vi "rs3 set multi options.vi"(4 "laser on/off":bool, 6 "autoexposure":bool, 7 "Laser power, mW (0-360)":sgl, 8 "error in (no error)":errorcluster, 9 "Gain(16-248)":sgl=16.0, 10 "Exposure, us":sgl=33000.0, 11 "Sensor in":u64) -> (0 "error out":errorcluster, 2 "Set Option error":string, 3 "Sensor out":u64)   [LabVIEW 2017, in "libRealSense3.lvlib"]
doc: "Sets the multiple device options. \n \nINPUT:\nExposure The manual exposure of the SENSOR, in microseconds\nGain The gain of the sensor from 16-248. For best results for depth keep this as low as possible\nLaser power The power of the projector in mW.\nLaser on/off Turns projector on/off.\nautoexposure Turns on the autoexplosure function which will automatically adjust gain and exposure. To change the setpoint it is possible to use the VIs that change the ROI (region of intested) as well as the SETPOINT for the autoexposure function. \n \nOutput:\nerror if non-null, receives any error that occurs during this call, otherwise, errors are ignored"
uses:
  <vilib>/addons/RealSense/libRealSense3.lvlib
panel:
  # "RS2_OPTION_BACKLIGHT_COMPENSATION                     , /**< Enable / disable color backlight compensation*/\n    RS2_OPTION_BRIGHTNESS                                 , /**< Color image brightness*/\n    RS2_OPTION_CONTRAST                                   , /**< Color image contrast*/\n    RS2_OPTION_EXPOSURE                                   , /**< Controls exposure time of color camera. Setting any value will disable auto exposure*/\n    RS2_OPTION_GAIN                                       , /**< Color image gain*/\n    RS2_OPTION_GAMMA                                      , /**< Color image gamma setting*/\n    RS2_OPTION_HUE                                        , /**< Color image hue*/\n    RS2_OPTION_SATURATION                                 , /**< Color image saturation setting*/\n    RS2_OPTION_SHARPNESS                                  , /**< Color image sharpness setting*/\n    RS2_OPTION_WHITE_BALANCE                              , /**< Controls white balance of color image. Setting any value will disable auto white balance*/\n    RS2_OPTION_ENABLE_AUTO_EXPOSURE                       , /**< Enable / disable color image auto-exposure*/\n    RS2_OPTION_ENABLE_AUTO_WHITE_BALANCE                  , /**< Enable / disable color image auto-white-balance*/\n    RS2_OPTION_VISUAL_PRESET                              , /**< Provide access to several recommend sets of option presets for the depth camera */\n    RS2_OPTION_LASER_POWER                                , /**< Power of the F200 / SR300 projector, with 0 meaning projector off*/\n    RS2_OPTION_ACCURACY                                   , /**< Set the number of patterns projected per frame. The higher the accuracy value the more patterns projected. Increasing the number of patterns help to achieve better accuracy. Note that this control is affecting the Depth FPS */\n    RS2_OPTION_MOTION_RANGE                               , /**< Motion vs. Range trade-off, with lower values allowing for better motion sensitivity and higher values allowing for better depth range*/\n    RS2_OPTION_FILTER_OPTION                              , /**< Set the filter to apply to each depth frame. Each one of the filter is optimized per the application requirements*/\n    RS2_OPTION_CONFIDENCE_THRESHOLD                       , /**< The confidence level threshold used by the Depth algorithm pipe to set whether a pixel will get a valid range or will be marked with invalid range*/\n    RS2_OPTION_EMITTER_ENABLED                            , /**< Laser Emitter enabled */\n    RS2_OPTION_FRAMES_QUEUE_SIZE                          , /**< Number of frames the user is allowed to keep per stream. Trying to hold-on to more frames will cause frame-drops.*/\n    RS2_OPTION_TOTAL_FRAME_DROPS                          , /**< Total number of detected frame drops from all streams */\n    RS2_OPTION_AUTO_EXPOSURE_MODE                         , /**< Auto-Exposure modes: Static, Anti-Flicker and Hybrid */\n    RS2_OPTION_AUTO_EXPOSURE_ANTIFLICKER_RATE             , /**< Auto-Exposure anti-flicker rate, can be 50 or 60 Hz */\n    RS2_OPTION_ASIC_TEMPERATURE                           , /**< Current Asic Temperature */\n    RS2_OPTION_ERROR_POLLING_ENABLED                      , /**< disable error handling */\n    RS2_OPTION_PROJECTOR_TEMPERATURE                      , /**< Current Projector Temperature */\n    RS2_OPTION_OUTPUT_TRIGGER_ENABLED                     , /**< Enable / disable trigger to be outputed from the camera to any external device on every depth frame */\n    RS2_OPTION_MOTION_MODULE_TEMPERATURE                  , /**< Current Motion-Module Temperature */\n    RS2_OPTION_COUNT                                      , /**< Number of enumeration values. Not a valid input: intended to be used in for-loops. */"
  # "RS3 Set Multi Device Option"
  # "(C) 2017 Intel Corp.,  AGJ"
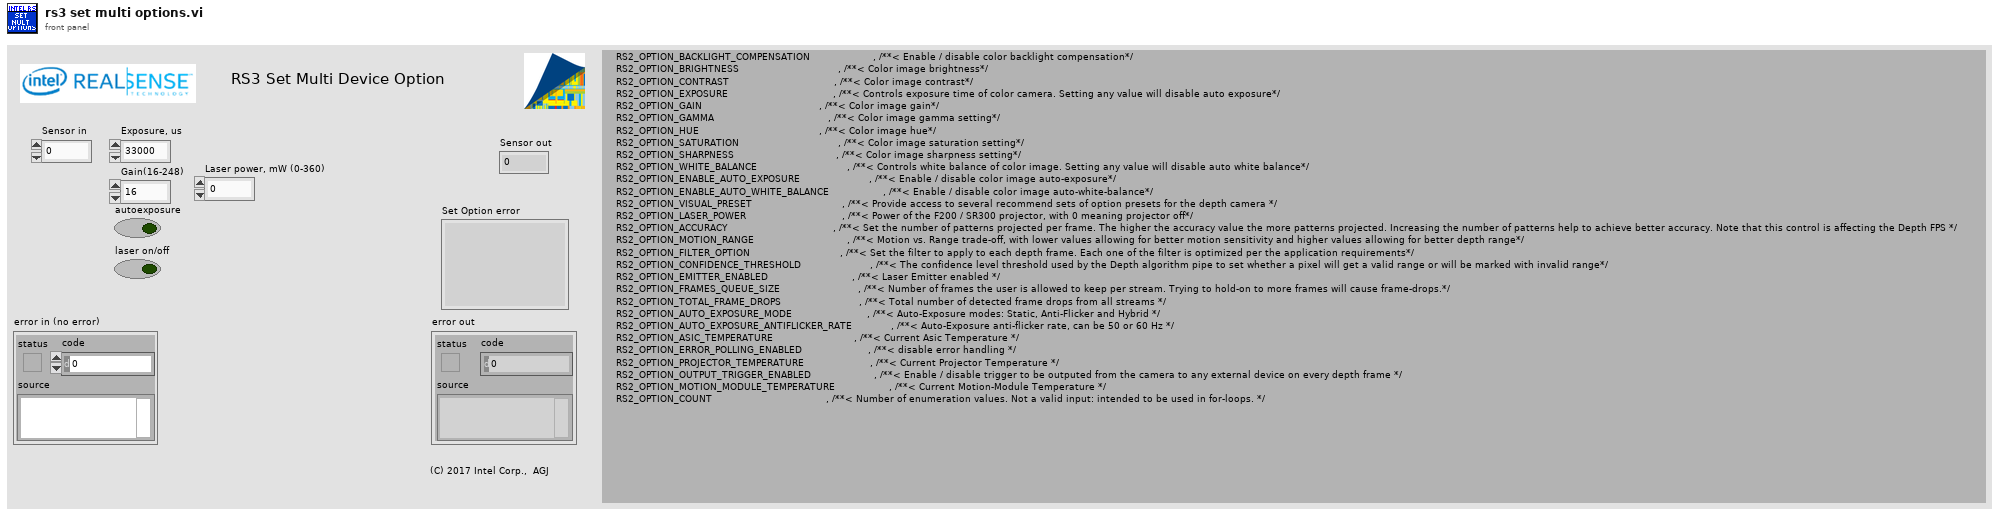
[diagram p1: front panel]
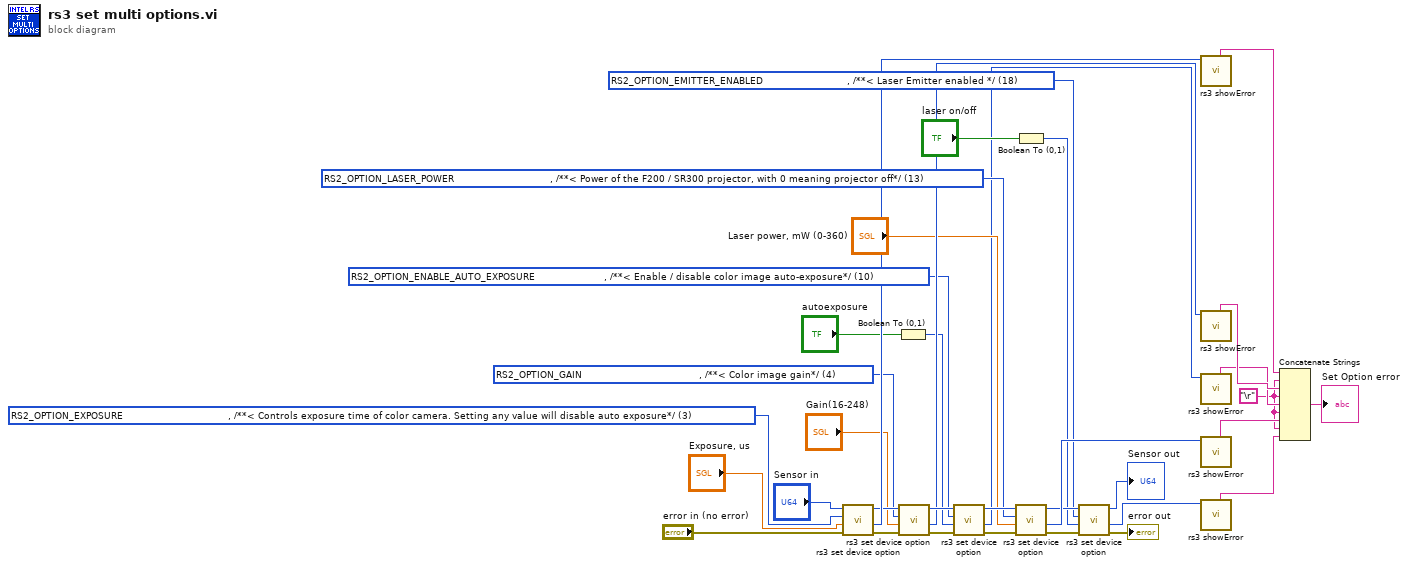
[diagram p0: block diagram]
diagram:
  w2 = u16 10 items=["    RS2_OPTION_BACKLIGHT_COMPENSATION                     , /**< Enable / disable color backlight compensation*/", "    RS2_OPTION_BRIGHTNESS                                 , /**< Color image brightness*/", "    RS2_OPTION_CONTRAST                                   , /**< Color image contrast*/", "    RS2_OPTION_EXPOSURE                                   , /**< Controls exposure time of color camera. Setting any value will disable auto exposure*/", "    RS2_OPTION_GAIN                                       , /**< Color image gain*/", "    RS2_OPTION_GAMMA                                      , /**< Color image gamma setting*/", "    RS2_OPTION_HUE                                        , /**< Color image hue*/", "    RS2_OPTION_SATURATION                                 , /**< Color image saturation setting*/", "    RS2_OPTION_SHARPNESS                                  , /**< Color image sharpness setting*/", "    RS2_OPTION_WHITE_BALANCE                              , /**< Controls white balance of color image. Setting any value will disable auto white balance*/", "    RS2_OPTION_ENABLE_AUTO_EXPOSURE                       , /**< Enable / disable color image auto-exposure*/", "    RS2_OPTION_ENABLE_AUTO_WHITE_BALANCE                  , /**< Enable / disable color image auto-white-balance*/", "    RS2_OPTION_VISUAL_PRESET                              , /**< Provide access to several recommend sets of option presets for the depth camera */", "    RS2_OPTION_LASER_POWER                                , /**< Power of the F200 / SR300 projector, with 0 meaning projector off*/", "    RS2_OPTION_ACCURACY                                   , /**< Set the number of patterns projected per frame. The higher the accuracy value the more patterns projected. Increasing the number of patterns help to achieve better accuracy. Note that this c", "    RS2_OPTION_MOTION_RANGE                               , /**< Motion vs. Range trade-off, with lower values allowing for better motion sensitivity and higher values allowing for better depth range*/", "    RS2_OPTION_FILTER_OPTION                              , /**< Set the filter to apply to each depth frame. Each one of the filter is optimized per the application requirements*/", "    RS2_OPTION_CONFIDENCE_THRESHOLD                       , /**< The confidence level threshold used by the Depth algorithm pipe to set whether a pixel will get a valid range or will be marked with invalid range*/", "    RS2_OPTION_EMITTER_ENABLED                            , /**< Laser Emitter enabled */", "    RS2_OPTION_FRAMES_QUEUE_SIZE                          , /**< Number of frames the user is allowed to keep per stream. Trying to hold-on to more frames will cause frame-drops.*/", "    RS2_OPTION_TOTAL_FRAME_DROPS                          , /**< Total number of detected frame drops from all streams */", "    RS2_OPTION_AUTO_EXPOSURE_MODE                         , /**< Auto-Exposure modes: Static, Anti-Flicker and Hybrid */", "    RS2_OPTION_POWER_LINE_FREQUENCY                       , /**< Power Line Frequency control for anti-flickering Off/50Hz/60Hz/Auto */", "    RS2_OPTION_ASIC_TEMPERATURE                           , /**< Current Asic Temperature */", "    RS2_OPTION_ERROR_POLLING_ENABLED                      , /**< disable error handling */", "    RS2_OPTION_PROJECTOR_TEMPERATURE                      , /**< Current Projector Temperature */", "    RS2_OPTION_OUTPUT_TRIGGER_ENABLED                     , /**< Enable / disable trigger to be outputed from the camera to any external device on every depth frame */", "    RS2_OPTION_MOTION_MODULE_TEMPERATURE                  , /**< Current Motion-Module Temperature */", "    RS2_OPTION_DEPTH_UNITS                                , /**< Number of meters represented by a single depth unit */", "    RS2_OPTION_ENABLE_MOTION_CORRECTION                   , /**< Enable/Disable automatic correction of the motion data */", "    RS2_OPTION_AUTO_EXPOSURE_PRIORITY                     , /**< Allows sensor to dynamically ajust the frame rate depending on lighting conditions */", "    RS2_OPTION_COUNT                                      , /**< Number of enumeration values. Not a valid input: intended to be used in for-loops. */"] ("RS Option")
  w5 = u16 13 items=["    RS2_OPTION_BACKLIGHT_COMPENSATION                     , /**< Enable / disable color backlight compensation*/", "    RS2_OPTION_BRIGHTNESS                                 , /**< Color image brightness*/", "    RS2_OPTION_CONTRAST                                   , /**< Color image contrast*/", "    RS2_OPTION_EXPOSURE                                   , /**< Controls exposure time of color camera. Setting any value will disable auto exposure*/", "    RS2_OPTION_GAIN                                       , /**< Color image gain*/", "    RS2_OPTION_GAMMA                                      , /**< Color image gamma setting*/", "    RS2_OPTION_HUE                                        , /**< Color image hue*/", "    RS2_OPTION_SATURATION                                 , /**< Color image saturation setting*/", "    RS2_OPTION_SHARPNESS                                  , /**< Color image sharpness setting*/", "    RS2_OPTION_WHITE_BALANCE                              , /**< Controls white balance of color image. Setting any value will disable auto white balance*/", "    RS2_OPTION_ENABLE_AUTO_EXPOSURE                       , /**< Enable / disable color image auto-exposure*/", "    RS2_OPTION_ENABLE_AUTO_WHITE_BALANCE                  , /**< Enable / disable color image auto-white-balance*/", "    RS2_OPTION_VISUAL_PRESET                              , /**< Provide access to several recommend sets of option presets for the depth camera */", "    RS2_OPTION_LASER_POWER                                , /**< Power of the F200 / SR300 projector, with 0 meaning projector off*/", "    RS2_OPTION_ACCURACY                                   , /**< Set the number of patterns projected per frame. The higher the accuracy value the more patterns projected. Increasing the number of patterns help to achieve better accuracy. Note that this c", "    RS2_OPTION_MOTION_RANGE                               , /**< Motion vs. Range trade-off, with lower values allowing for better motion sensitivity and higher values allowing for better depth range*/", "    RS2_OPTION_FILTER_OPTION                              , /**< Set the filter to apply to each depth frame. Each one of the filter is optimized per the application requirements*/", "    RS2_OPTION_CONFIDENCE_THRESHOLD                       , /**< The confidence level threshold used by the Depth algorithm pipe to set whether a pixel will get a valid range or will be marked with invalid range*/", "    RS2_OPTION_EMITTER_ENABLED                            , /**< Laser Emitter enabled */", "    RS2_OPTION_FRAMES_QUEUE_SIZE                          , /**< Number of frames the user is allowed to keep per stream. Trying to hold-on to more frames will cause frame-drops.*/", "    RS2_OPTION_TOTAL_FRAME_DROPS                          , /**< Total number of detected frame drops from all streams */", "    RS2_OPTION_AUTO_EXPOSURE_MODE                         , /**< Auto-Exposure modes: Static, Anti-Flicker and Hybrid */", "    RS2_OPTION_POWER_LINE_FREQUENCY                       , /**< Power Line Frequency control for anti-flickering Off/50Hz/60Hz/Auto */", "    RS2_OPTION_ASIC_TEMPERATURE                           , /**< Current Asic Temperature */", "    RS2_OPTION_ERROR_POLLING_ENABLED                      , /**< disable error handling */", "    RS2_OPTION_PROJECTOR_TEMPERATURE                      , /**< Current Projector Temperature */", "    RS2_OPTION_OUTPUT_TRIGGER_ENABLED                     , /**< Enable / disable trigger to be outputed from the camera to any external device on every depth frame */", "    RS2_OPTION_MOTION_MODULE_TEMPERATURE                  , /**< Current Motion-Module Temperature */", "    RS2_OPTION_DEPTH_UNITS                                , /**< Number of meters represented by a single depth unit */", "    RS2_OPTION_ENABLE_MOTION_CORRECTION                   , /**< Enable/Disable automatic correction of the motion data */", "    RS2_OPTION_AUTO_EXPOSURE_PRIORITY                     , /**< Allows sensor to dynamically ajust the frame rate depending on lighting conditions */", "    RS2_OPTION_COUNT                                      , /**< Number of enumeration values. Not a valid input: intended to be used in for-loops. */"] ("RS Option")
  w7 = u16 18 items=["    RS2_OPTION_BACKLIGHT_COMPENSATION                     , /**< Enable / disable color backlight compensation*/", "    RS2_OPTION_BRIGHTNESS                                 , /**< Color image brightness*/", "    RS2_OPTION_CONTRAST                                   , /**< Color image contrast*/", "    RS2_OPTION_EXPOSURE                                   , /**< Controls exposure time of color camera. Setting any value will disable auto exposure*/", "    RS2_OPTION_GAIN                                       , /**< Color image gain*/", "    RS2_OPTION_GAMMA                                      , /**< Color image gamma setting*/", "    RS2_OPTION_HUE                                        , /**< Color image hue*/", "    RS2_OPTION_SATURATION                                 , /**< Color image saturation setting*/", "    RS2_OPTION_SHARPNESS                                  , /**< Color image sharpness setting*/", "    RS2_OPTION_WHITE_BALANCE                              , /**< Controls white balance of color image. Setting any value will disable auto white balance*/", "    RS2_OPTION_ENABLE_AUTO_EXPOSURE                       , /**< Enable / disable color image auto-exposure*/", "    RS2_OPTION_ENABLE_AUTO_WHITE_BALANCE                  , /**< Enable / disable color image auto-white-balance*/", "    RS2_OPTION_VISUAL_PRESET                              , /**< Provide access to several recommend sets of option presets for the depth camera */", "    RS2_OPTION_LASER_POWER                                , /**< Power of the F200 / SR300 projector, with 0 meaning projector off*/", "    RS2_OPTION_ACCURACY                                   , /**< Set the number of patterns projected per frame. The higher the accuracy value the more patterns projected. Increasing the number of patterns help to achieve better accuracy. Note that this c", "    RS2_OPTION_MOTION_RANGE                               , /**< Motion vs. Range trade-off, with lower values allowing for better motion sensitivity and higher values allowing for better depth range*/", "    RS2_OPTION_FILTER_OPTION                              , /**< Set the filter to apply to each depth frame. Each one of the filter is optimized per the application requirements*/", "    RS2_OPTION_CONFIDENCE_THRESHOLD                       , /**< The confidence level threshold used by the Depth algorithm pipe to set whether a pixel will get a valid range or will be marked with invalid range*/", "    RS2_OPTION_EMITTER_ENABLED                            , /**< Laser Emitter enabled */", "    RS2_OPTION_FRAMES_QUEUE_SIZE                          , /**< Number of frames the user is allowed to keep per stream. Trying to hold-on to more frames will cause frame-drops.*/", "    RS2_OPTION_TOTAL_FRAME_DROPS                          , /**< Total number of detected frame drops from all streams */", "    RS2_OPTION_AUTO_EXPOSURE_MODE                         , /**< Auto-Exposure modes: Static, Anti-Flicker and Hybrid */", "    RS2_OPTION_POWER_LINE_FREQUENCY                       , /**< Power Line Frequency control for anti-flickering Off/50Hz/60Hz/Auto */", "    RS2_OPTION_ASIC_TEMPERATURE                           , /**< Current Asic Temperature */", "    RS2_OPTION_ERROR_POLLING_ENABLED                      , /**< disable error handling */", "    RS2_OPTION_PROJECTOR_TEMPERATURE                      , /**< Current Projector Temperature */", "    RS2_OPTION_OUTPUT_TRIGGER_ENABLED                     , /**< Enable / disable trigger to be outputed from the camera to any external device on every depth frame */", "    RS2_OPTION_MOTION_MODULE_TEMPERATURE                  , /**< Current Motion-Module Temperature */", "    RS2_OPTION_DEPTH_UNITS                                , /**< Number of meters represented by a single depth unit */", "    RS2_OPTION_ENABLE_MOTION_CORRECTION                   , /**< Enable/Disable automatic correction of the motion data */", "    RS2_OPTION_AUTO_EXPOSURE_PRIORITY                     , /**< Allows sensor to dynamically ajust the frame rate depending on lighting conditions */", "    RS2_OPTION_COUNT                                      , /**< Number of enumeration values. Not a valid input: intended to be used in for-loops. */"] ("RS Option")
  w13 = u16 4 items=["    RS2_OPTION_BACKLIGHT_COMPENSATION                     , /**< Enable / disable color backlight compensation*/", "    RS2_OPTION_BRIGHTNESS                                 , /**< Color image brightness*/", "    RS2_OPTION_CONTRAST                                   , /**< Color image contrast*/", "    RS2_OPTION_EXPOSURE                                   , /**< Controls exposure time of color camera. Setting any value will disable auto exposure*/", "    RS2_OPTION_GAIN                                       , /**< Color image gain*/", "    RS2_OPTION_GAMMA                                      , /**< Color image gamma setting*/", "    RS2_OPTION_HUE                                        , /**< Color image hue*/", "    RS2_OPTION_SATURATION                                 , /**< Color image saturation setting*/", "    RS2_OPTION_SHARPNESS                                  , /**< Color image sharpness setting*/", "    RS2_OPTION_WHITE_BALANCE                              , /**< Controls white balance of color image. Setting any value will disable auto white balance*/", "    RS2_OPTION_ENABLE_AUTO_EXPOSURE                       , /**< Enable / disable color image auto-exposure*/", "    RS2_OPTION_ENABLE_AUTO_WHITE_BALANCE                  , /**< Enable / disable color image auto-white-balance*/", "    RS2_OPTION_VISUAL_PRESET                              , /**< Provide access to several recommend sets of option presets for the depth camera */", "    RS2_OPTION_LASER_POWER                                , /**< Power of the F200 / SR300 projector, with 0 meaning projector off*/", "    RS2_OPTION_ACCURACY                                   , /**< Set the number of patterns projected per frame. The higher the accuracy value the more patterns projected. Increasing the number of patterns help to achieve better accuracy. Note that this c", "    RS2_OPTION_MOTION_RANGE                               , /**< Motion vs. Range trade-off, with lower values allowing for better motion sensitivity and higher values allowing for better depth range*/", "    RS2_OPTION_FILTER_OPTION                              , /**< Set the filter to apply to each depth frame. Each one of the filter is optimized per the application requirements*/", "    RS2_OPTION_CONFIDENCE_THRESHOLD                       , /**< The confidence level threshold used by the Depth algorithm pipe to set whether a pixel will get a valid range or will be marked with invalid range*/", "    RS2_OPTION_EMITTER_ENABLED                            , /**< Laser Emitter enabled */", "    RS2_OPTION_FRAMES_QUEUE_SIZE                          , /**< Number of frames the user is allowed to keep per stream. Trying to hold-on to more frames will cause frame-drops.*/", "    RS2_OPTION_TOTAL_FRAME_DROPS                          , /**< Total number of detected frame drops from all streams */", "    RS2_OPTION_AUTO_EXPOSURE_MODE                         , /**< Auto-Exposure modes: Static, Anti-Flicker and Hybrid */", "    RS2_OPTION_POWER_LINE_FREQUENCY                       , /**< Power Line Frequency control for anti-flickering Off/50Hz/60Hz/Auto */", "    RS2_OPTION_ASIC_TEMPERATURE                           , /**< Current Asic Temperature */", "    RS2_OPTION_ERROR_POLLING_ENABLED                      , /**< disable error handling */", "    RS2_OPTION_PROJECTOR_TEMPERATURE                      , /**< Current Projector Temperature */", "    RS2_OPTION_OUTPUT_TRIGGER_ENABLED                     , /**< Enable / disable trigger to be outputed from the camera to any external device on every depth frame */", "    RS2_OPTION_MOTION_MODULE_TEMPERATURE                  , /**< Current Motion-Module Temperature */", "    RS2_OPTION_DEPTH_UNITS                                , /**< Number of meters represented by a single depth unit */", "    RS2_OPTION_ENABLE_MOTION_CORRECTION                   , /**< Enable/Disable automatic correction of the motion data */", "    RS2_OPTION_AUTO_EXPOSURE_PRIORITY                     , /**< Allows sensor to dynamically ajust the frame rate depending on lighting conditions */", "    RS2_OPTION_COUNT                                      , /**< Number of enumeration values. Not a valid input: intended to be used in for-loops. */"] ("RS Option")
  w21 = u16 3 items=["    RS2_OPTION_BACKLIGHT_COMPENSATION                     , /**< Enable / disable color backlight compensation*/", "    RS2_OPTION_BRIGHTNESS                                 , /**< Color image brightness*/", "    RS2_OPTION_CONTRAST                                   , /**< Color image contrast*/", "    RS2_OPTION_EXPOSURE                                   , /**< Controls exposure time of color camera. Setting any value will disable auto exposure*/", "    RS2_OPTION_GAIN                                       , /**< Color image gain*/", "    RS2_OPTION_GAMMA                                      , /**< Color image gamma setting*/", "    RS2_OPTION_HUE                                        , /**< Color image hue*/", "    RS2_OPTION_SATURATION                                 , /**< Color image saturation setting*/", "    RS2_OPTION_SHARPNESS                                  , /**< Color image sharpness setting*/", "    RS2_OPTION_WHITE_BALANCE                              , /**< Controls white balance of color image. Setting any value will disable auto white balance*/", "    RS2_OPTION_ENABLE_AUTO_EXPOSURE                       , /**< Enable / disable color image auto-exposure*/", "    RS2_OPTION_ENABLE_AUTO_WHITE_BALANCE                  , /**< Enable / disable color image auto-white-balance*/", "    RS2_OPTION_VISUAL_PRESET                              , /**< Provide access to several recommend sets of option presets for the depth camera */", "    RS2_OPTION_LASER_POWER                                , /**< Power of the F200 / SR300 projector, with 0 meaning projector off*/", "    RS2_OPTION_ACCURACY                                   , /**< Set the number of patterns projected per frame. The higher the accuracy value the more patterns projected. Increasing the number of patterns help to achieve better accuracy. Note that this c", "    RS2_OPTION_MOTION_RANGE                               , /**< Motion vs. Range trade-off, with lower values allowing for better motion sensitivity and higher values allowing for better depth range*/", "    RS2_OPTION_FILTER_OPTION                              , /**< Set the filter to apply to each depth frame. Each one of the filter is optimized per the application requirements*/", "    RS2_OPTION_CONFIDENCE_THRESHOLD                       , /**< The confidence level threshold used by the Depth algorithm pipe to set whether a pixel will get a valid range or will be marked with invalid range*/", "    RS2_OPTION_EMITTER_ENABLED                            , /**< Laser Emitter enabled */", "    RS2_OPTION_FRAMES_QUEUE_SIZE                          , /**< Number of frames the user is allowed to keep per stream. Trying to hold-on to more frames will cause frame-drops.*/", "    RS2_OPTION_TOTAL_FRAME_DROPS                          , /**< Total number of detected frame drops from all streams */", "    RS2_OPTION_AUTO_EXPOSURE_MODE                         , /**< Auto-Exposure modes: Static, Anti-Flicker and Hybrid */", "    RS2_OPTION_POWER_LINE_FREQUENCY                       , /**< Power Line Frequency control for anti-flickering Off/50Hz/60Hz/Auto */", "    RS2_OPTION_ASIC_TEMPERATURE                           , /**< Current Asic Temperature */", "    RS2_OPTION_ERROR_POLLING_ENABLED                      , /**< disable error handling */", "    RS2_OPTION_PROJECTOR_TEMPERATURE                      , /**< Current Projector Temperature */", "    RS2_OPTION_OUTPUT_TRIGGER_ENABLED                     , /**< Enable / disable trigger to be outputed from the camera to any external device on every depth frame */", "    RS2_OPTION_MOTION_MODULE_TEMPERATURE                  , /**< Current Motion-Module Temperature */", "    RS2_OPTION_DEPTH_UNITS                                , /**< Number of meters represented by a single depth unit */", "    RS2_OPTION_ENABLE_MOTION_CORRECTION                   , /**< Enable/Disable automatic correction of the motion data */", "    RS2_OPTION_AUTO_EXPOSURE_PRIORITY                     , /**< Allows sensor to dynamically ajust the frame rate depending on lighting conditions */", "    RS2_OPTION_COUNT                                      , /**< Number of enumeration values. Not a valid input: intended to be used in for-loops. */"] ("RS Option")
  w23 = "\r"
  n1 = call <vilib>:"rs3 set device option.vi"("error in (no error)"="error in (no error)", "value"="Exposure, us", "RS Option"=w21, "Sensor in"="Sensor in") -> ("error out"=w32:errorcluster, "error"=w33:u64, "Sensor out"=w19:u64)  [unwired: 5 in]
  n2 = Boolean To (0,1)(Boolean="autoexposure") -> (0, 1=w3:i16)
  n3 = call <vilib>:"rs3 set device option.vi"("error in (no error)"=w32, "value"="Gain(16-248)", "RS Option"=w13, "Sensor in"=w19) -> ("error out"=w31:errorcluster, "error"=w8:u64, "Sensor out"=w14:u64)  [unwired: 5 in]
  n4 = call <vilib>:"rs3 set device option.vi"("error in (no error)"=w31, "value"=w3, "RS Option"=w2, "Sensor in"=w14) -> ("error out"=w30:errorcluster, "error"=w1:u64, "Sensor out"=w15:u64)  [unwired: 5 in]
  n5 = Boolean To (0,1)(Boolean="laser on/off") -> (0, 1=w6:i16)
  n6 = call <vilib>:"rs3 set device option.vi"("error in (no error)"=w30, "value"="Laser power, mW (0-360)", "RS Option"=w5, "Sensor in"=w15) -> ("error out"=w29:errorcluster, "error"=w18:u64, "Sensor out"=w16:u64)  [unwired: 5 in]
  n7 = call <vilib>:"rs3 set device option.vi"("error in (no error)"=w29, "value"=w6, "RS Option"=w7, "Sensor in"=w16) -> ("error out"=→"error out":errorcluster, "error"=w17:u64, "Sensor out"=→"Sensor out":u64)  [unwired: 5 in]
  n8 = call <vilib>:"rs3 showError.vi"("error"=w33) -> ("Error summary"=w27:string)  [unwired: 6 in, 4 out]
  n9 = call <vilib>:"rs3 showError.vi"("error"=w8) -> ("Error summary"=w26:string)  [unwired: 6 in, 4 out]
  n10 = call <vilib>:"rs3 showError.vi"("error"=w1) -> ("Error summary"=w25:string)  [unwired: 6 in, 4 out]
  n11 = call <vilib>:"rs3 showError.vi"("error"=w18) -> ("Error summary"=w24:string)  [unwired: 6 in, 4 out]
  n12 = call <vilib>:"rs3 showError.vi"("error"=w17) -> ("Error summary"=w22:string)  [unwired: 6 in, 4 out]
  n13 = Concatenate Strings(w27, w23, w26, w23, w25, w23, w24, w23, w22) -> (→"Set Option error":string)
